vi "Contour Line_Find Connected Contour Points.vi"(8 "height":dbl, 10 "Intersected Edges":T3(array[cluster]), 11 "Contour Points":cluster{"x":dbl, "y":dbl}[](array[cluster])) -> (3 "Contour Line":T1)   [LabVIEW 2020, in "NI_AAL_Geometry.lvlib"]
uses:
  <vilib>/Analysis/NI_AAL_Geometry.lvlib
  <vilib>/Analysis/geometry.llb/Contour Lines Control.ctl
  <vilib>/Analysis/geometry.llb/Contour Line Segment.ctl
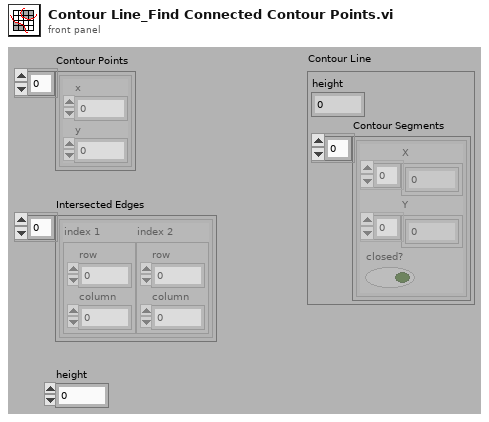
[diagram p1: front panel]
types:
  T1 = typedef "NI_AAL_Geometry.lvlib/Contour Lines Control.ctl" = cluster{"height":dbl, "Contour Segments":T2[]}
  T2 = typedef "NI_AAL_Geometry.lvlib/Contour Line Segment.ctl" = cluster{"X":dbl[], "Y":dbl[], "closed?":bool}
  T3 = cluster{"index 1":cluster{"row":i32, "column":i32}, "index 2":cluster{"row":i32, "column":i32}}[]
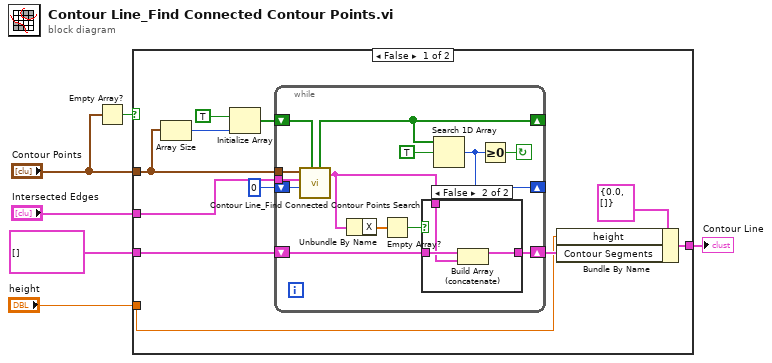
[diagram p0: block diagram]
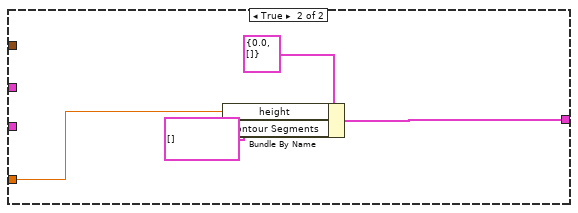
[diagram p3: hidden frame]
diagram:
  n1 = Empty Array?(array="Contour Points") -> (empty?=w4:bool)
  n2 = case shown="False" w4 {
    tunnel: "Contour Points" -> [w17 _]
    tunnel: "Intersected Edges" -> [w13 _]
    tunnel: T2[] [] -> [w11 _]
    tunnel: "height" -> [w8 w36]
    tunnel: [w7 w37] -> w1
    frame False {
      n3 = Array Size(array=w17) -> (size(s)=w16:i32)
      n4 = Initialize Array(TRUE, w16) -> (w12:bool[])
      n5 = while {
        shift-right: [w24] -> _
        shift-left: 0 -> [w27]
        tunnel: w17 -> [w30]
        tunnel: w13 -> [w28]
        shift-right: [w26] -> _
        shift-left: w12 -> [w29]
        shift-right: [w22] -> w10
        shift-left: w11 -> [w21]
        stop <- w23 continue-if-true
        n6 = call <vilib>:"Contour Line_Find Connected Contour Points Search.vi"("Stack In"=w29, "index"=w27, "Intersected Edges"=w28, "Contour Points"=w30) -> ("Contour Segment"=w20:T2, "Stack Out"=w26:bool[])  [unwired: 1 in, 5 out]
        n7 = Unbundle By Name(w20) -> ("X"=w19:dbl[])
        n8 = Empty Array?(array=w19) -> (empty?=w18:bool)
        n9 = case shown="False" w18 {
          tunnel: [w31 w34] -> w22
          tunnel: w21 -> [w31 w33]
          tunnel: w20 -> [_ w32]
          frame True {
          }
          frame False {
            n10 = Build Array (concatenate)(w33, w32) -> (w34:T2[])
          }
        }
        n11 = Search 1D Array(1D array=w26, element=TRUE) -> (index of element=w24:i32)  [unwired: 1 out]
        n12 = Greater Or Equal To 0?(x=w24) -> (x >= 0?=w23:bool)
      }
      n13 = Bundle By Name(cluster=T1 {"height"=0.0, "Contour Segments"=[]} ("Contour Line"), "height"=w8, "Contour Segments"=w10) -> (w7:T1)
    }
    frame True {
      n14 = Bundle By Name(cluster=T1 {"height"=0.0, "Contour Segments"=[]} ("Contour Line"), "height"=w36, "Contour Segments"=T2[] [] ("Segments")) -> (w37:T1)
    }
  }
  "Contour Line" <- w1
